vi "FGV_data_exchange.vi"(7 "FGV states":T1, 8 "error in (no error)":errorcluster) -> (0 "error out":errorcluster, 3 "main_cycle_queue":T2)   [LabVIEW 2020]
uses:
  data_exchange_fgv.ctl
  AppStates.ctl
  <vilib>/sound2/lvsound2.llb/Sound Output Task ID.ctl
  FGVstates.ctl
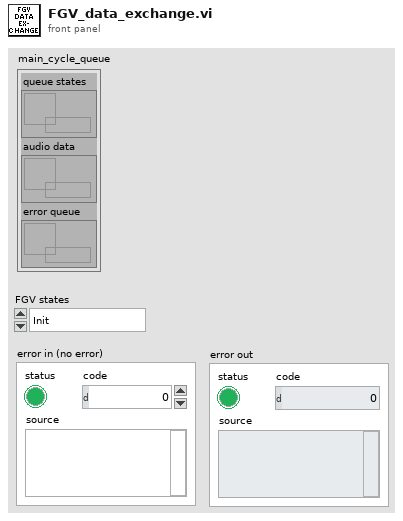
[diagram p1: front panel]
types:
  T1 = typedef "FGVstates.ctl" = enum16{"Init", "Set", "Get", "De-Init"}
  T2 = typedef "data_exchange_fgv.ctl" = cluster{"queue states":refnum<queue>, "audio data":refnum<queue>, "error queue":refnum<queue>}
  T3 = typedef "AppStates.ctl" = enum16{"Init", "Scan Music Dir", "Idle", "Playback", "Enqueue samples", "Pause playback", "Stop playback", "Exit"}
  T4 = typedef "Sound Output Task ID.ctl" = u32
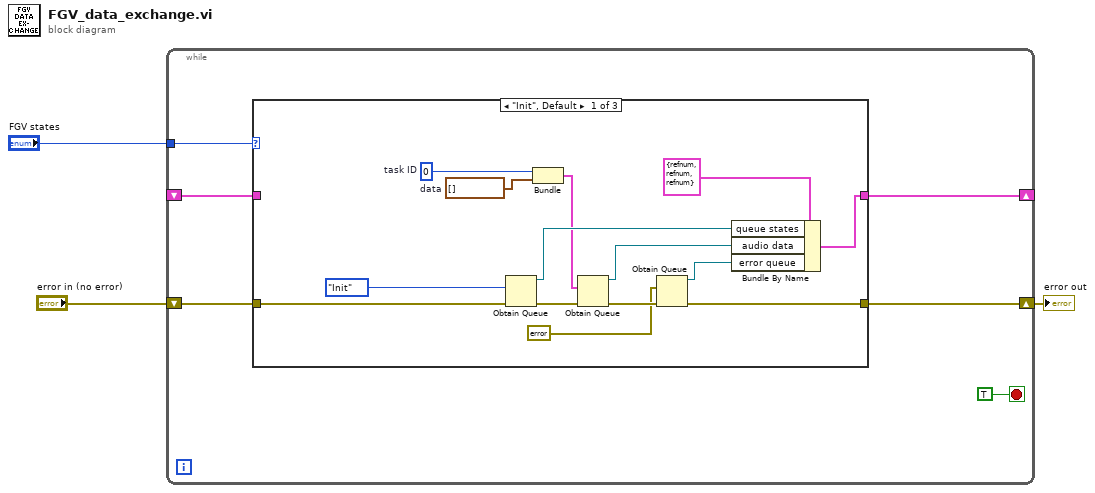
[diagram p0: block diagram]
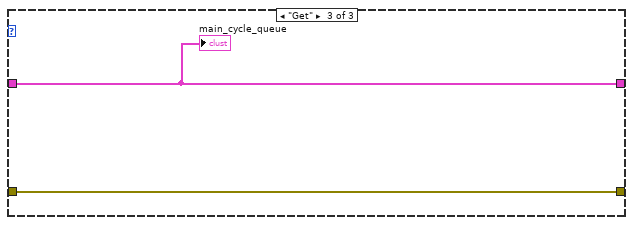
[diagram p3: hidden frame]
diagram:
  n1 = while {
    tunnel: "FGV states" -> [w8]
    shift-right: [w4] -> w1
    shift-left: "error in (no error)" -> [w6]
    shift-right: [w7] -> _
    shift-left: _ -> [w5]
    stop <- TRUE stop-if-true
    n2 = case shown="\"Init\", Default" w8 {
      tunnel: [w18 w24 w26] -> w7
      tunnel: w6 -> [w22 w25 w27]
      tunnel: w5 -> [_ w24 w26]
      tunnel: [w13 w25 w27] -> w4
      frame "Init", Default {
        w15 = T4 0  # task ID
        w17 = waveform(dbl)[] []  # data
        n3 = Obtain Queue(element data type=AppStates."Init" ("Application States"), error in (no error)=w22) -> (queue out=w21:refnum<queue>, error out=w20:errorcluster)  [unwired: 3 in, 1 out]
        n4 = Bundle("task ID"=w15, "data"=w17) -> (w16:cluster{"task ID":T4, "data":waveform(dbl)[]})  [unwired: 1 in]
        n5 = Obtain Queue(element data type=w16, error in (no error)=w20) -> (queue out=w14:refnum<queue>, error out=w12:errorcluster)  [unwired: 3 in, 1 out]
        n6 = Obtain Queue(element data type=errorcluster {"status"=FALSE, "code"=0, "source"=""} ("error constant"), error in (no error)=w12) -> (queue out=w10:refnum<queue>, error out=w13:errorcluster)  [unwired: 3 in, 1 out]
        n7 = Bundle By Name(cluster=T2 {"queue states"=refnum, "audio data"=refnum, "error queue"=refnum} ("main_cycle_queue 2"), "queue states"=w21, "audio data"=w14, "error queue"=w10) -> (w18:T2)
      }
      frame "Set" {
      }
      frame "Get" {
        "main_cycle_queue" <- w26
      }
    }
  }
  "error out" <- w1
